vi "template_reading.vi"() -> ()   [LabVIEW 2022 SP3]
panel:
  out "Counts":i32[](array[numeric])
  out "OVL":bool caption="LED ON : Over Rang Data"
  out "OLD":i32
  out "GN":i32 caption="Gate Number"
  out "DB":u32[](array[numeric])
  in  "Correction":bool=TRUE
  in  "RN":i32=100 caption="Set Gate Number"
  in  "IT":i32=100 caption="Set Gate Time (ms)"
  out "Handle Number":i32
  # "SN: 30430219"
  # "need to figure out how to do many counts and stuff"
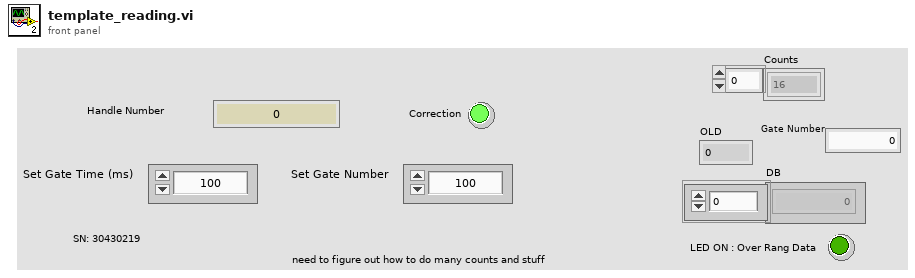
[diagram p1: front panel]
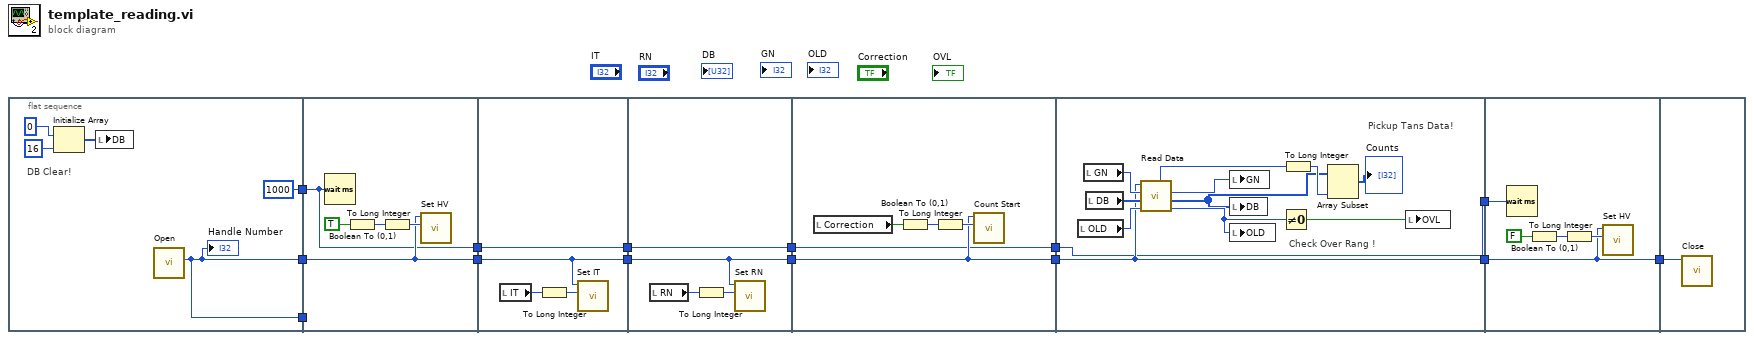
[diagram p0: block diagram]
diagram:
  n1 = flat-sequence {
    tunnel: [w16] -> w14
    tunnel: [w16] -> w8
    tunnel: [1000 ("次元サイズ")] -> w7
    tunnel: w14 -> [_]
    tunnel: [w21] -> w9
    tunnel: w8 -> [w21]
    tunnel: w7 -> [w20]
    tunnel: [w20] -> w6
    tunnel: [w26] -> w10
    tunnel: w9 -> [w26]
    tunnel: w6 -> [w25]
    tunnel: [w25] -> w5
    tunnel: [w30] -> w2
    tunnel: w10 -> [w30]
    tunnel: w5 -> [w29]
    tunnel: [w29] -> w1
    tunnel: [w34] -> w11
    tunnel: w2 -> [w34]
    tunnel: w1 -> [w33]
    tunnel: [w33] -> w4
    tunnel: [w39] -> w12
    tunnel: w11 -> [w39]
    tunnel: w4 -> [w38]
    tunnel: [w38] -> w3
    tunnel: [w51] -> w13
    tunnel: w12 -> [w51]
    tunnel: w3 -> [w50]
    tunnel: w13 -> [w55]
    frame #0 {
      # "DB Clear!"
      n2 = Initialize Array(u32 0, 16 ("次元サイズ")) -> (w19:u32[])
      n3 = local write "DB"(w19) -> ()
      n4 = call "Open.vi"() -> ("Handle Number"=w16:i32)  [unwired: 10 in, 1 out]
      "Handle Number" <- w16
    }
    frame #1 {
      n5 = Wait (ms)(milliseconds to wait=w20) -> ()  [unwired: 1 out]
      n6 = Boolean To (0,1)(Boolean=TRUE) -> (0, 1=w23:i16)
      n7 = To Long Integer(number=w23) -> (32bit integer=w24:i32)
      n8 = call "Set HV.vi"("HV"=w24, "handle"=w21) -> ()  [unwired: 8 in, 2 out]
    }
    frame #2 {
      n9 = local read "IT"() -> (w28:i32)
      n10 = To Long Integer(number=w28) -> (32bit integer=w27:i32)
      n11 = call "Set IT.vi"("IT"=w27, "handle"=w26) -> ()  [unwired: 8 in, 2 out]
    }
    frame #3 {
      n12 = local read "RN"() -> (w32:i32)
      n13 = To Long Integer(number=w32) -> (32bit integer=w31:i32)
      n14 = call "Set RN.vi"("RN"=w31, "handle"=w30) -> ()  [unwired: 8 in, 2 out]
    }
    frame #4 {
      n15 = local read "Correction"() -> (w37:bool)
      n16 = Boolean To (0,1)(Boolean=w37) -> (0, 1=w35:i16)
      n17 = To Long Integer(number=w35) -> (32bit integer=w36:i32)
      n18 = call "Count Start.vi"("Correction"=w36, "handle"=w34) -> ()  [unwired: 8 in, 2 out]
    }
    frame #5 {
      # "Check Over Rang !"
      # "Pickup Tans Data!"
      n19 = local read "OLD"() -> (w49:i32)
      n20 = local read "GN"() -> (w47:i32)
      n21 = local read "DB"() -> (w48:u32[])
      n22 = call "Read Data.vi"("OLD"=w49, "DataBuf"=w48, "GateNum"=w47, "handle"=w39) -> ("OLD out"=w42:i32, "DataBuf out"=w41:u32[], "GateNum out"=w43:i32, "function return"=w44:u32)  [unwired: 3 in, 1 out]
      n23 = local write "GN"(w43) -> ()
      n24 = local write "DB"(w41) -> ()
      n25 = local write "OLD"(w42) -> ()
      n26 = Not Equal To 0?(x=w42) -> (x != 0?=w46:bool)
      n27 = To Long Integer(number=w44) -> (32bit integer=w45:i32)
      n28 = Array Subset(array=w41, length=w45) -> (→"Counts":u32[])  [unwired: 1 in]
      n29 = local write "OVL"(w46) -> ()
    }
    frame #6 {
      n30 = Wait (ms)(milliseconds to wait=w50) -> ()  [unwired: 1 out]
      n31 = Boolean To (0,1)(Boolean=FALSE) -> (0, 1=w53:i16)
      n32 = To Long Integer(number=w53) -> (32bit integer=w54:i32)
      n33 = call "Set HV.vi"("HV"=w54, "handle"=w51) -> ()  [unwired: 8 in, 2 out]
    }
    frame #7 {
      n34 = call "Close.vi"("Handle"=w55) -> ()  [unwired: 9 in, 2 out]
    }
  }
